vi "Library Write Text File.vi"(0 "file path":path, 1 "convert eol (F)":bool, 7 "text to write":string, 11 "error in (no error)":errorcluster) -> (4 "dup path":path, 15 "error out":errorcluster)   [LabVIEW 2012]
doc: "Writes a text file with optional eol conversion."
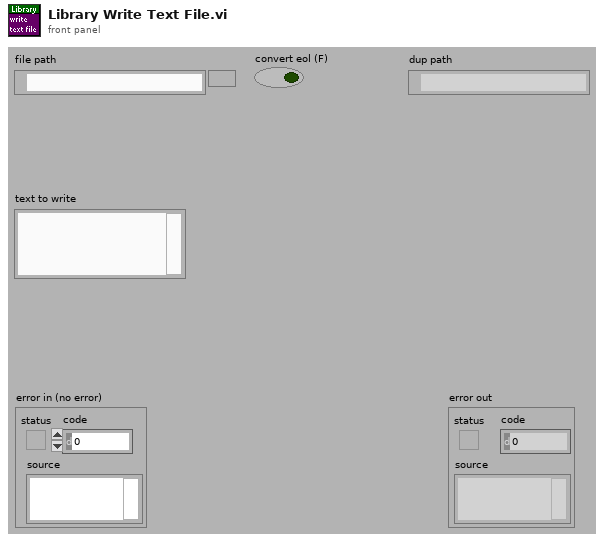
[diagram p1: front panel]
types:
  T1 = enum16{"deny read/write", "deny write-only", "deny none"}
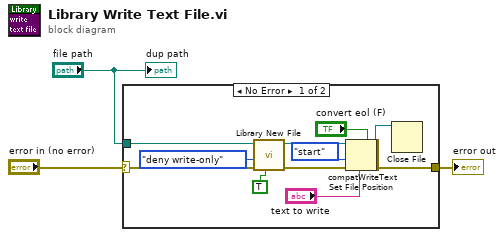
[diagram p0: block diagram]
diagram:
  n1 = case shown="No Error" "error in (no error)" {
    selector: "error in (no error)" -> [w15 w17]
    tunnel: [w16 w17] -> w3
    tunnel: "file path" -> [w6 _]
    frame No Error {
      n2 = call "Library New File.vi"("overwrite (F)"=TRUE, "error in (no error)"=w15, "deny mode (deny none)"=T1."deny write-only" ("deny mode (2)"), "file path"=w6) -> ("error out"=w11:errorcluster, "refnum"=w12:refnum<file>)  [unwired: 6 in]
      n3 = Set File Position(refnum=w12, from (0:start)=enum16{"start", "end", "current"}."start" ("pos mode (0:2)"), error in=w11) -> (refnum out=w5:refnum<file>, error out=w4:errorcluster)  [unwired: 1 in]
      n4 = call <vilib>:"compatWriteText.vi"("convert eol (F)"="convert eol (F)", "data"="text to write", "error in"=w4, "refnum"=w5) -> ("error out"=w16:errorcluster, "dup refnum"=w8:refnum<file>)  [unwired: 6 in]
      n5 = Close File(refnum=w8) -> ()  [unwired: 1 in, 2 out]
    }
    frame Error {
    }
  }
  "error out" <- w3
  "dup path" <- "file path"
